vi "GetCtrlRef (String).vi"(8 "error in (no error)":errorcluster, 10 "FP Control":string, 11 "FP Controls in":refnum<class "FP Controls.lvclass">) -> (0 "error out":errorcluster, 2 "Ctrl Ref":refnum<vi>, 3 "FP Controls out":refnum<class "FP Controls.lvclass">)   [LabVIEW 2012, in "Configuration Grandmaster.lvlib" / "FP Controls.lvclass"]
uses:
  FP Controls.lvclass
  FP Controls.lvclass/FP Controls.ctl
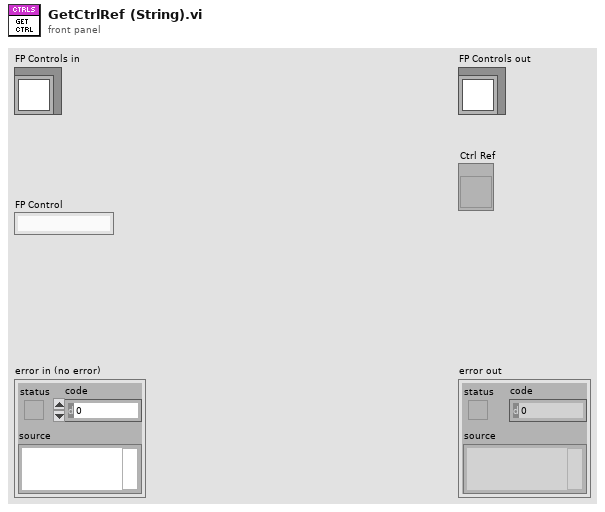
[diagram p1: front panel]
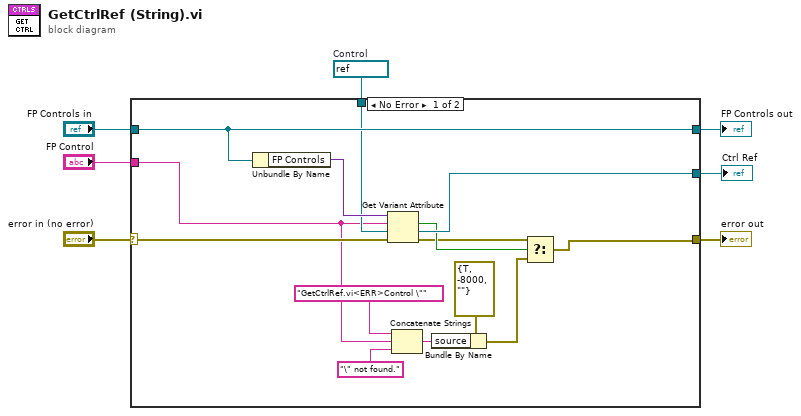
[diagram p0: block diagram]
diagram:
  w3 = refnum<vi> refnum  # Control
  n1 = case shown="No Error" "error in (no error)" {
    selector: "error in (no error)" -> [w9 w24]
    tunnel: [w15 w24] -> w6
    tunnel: [w21 w23] -> w4
    tunnel: "FP Controls in" -> [w21 w23]
    tunnel: w3 -> [w19 w22]
    tunnel: [w18 w22] -> w2
    tunnel: "FP Control" -> [w8 _]
    frame No Error {
      n2 = Unbundle By Name(w21) -> ("FP Controls"=w20:variant)
      n3 = Get Variant Attribute(Variant=w20, name=w8, default value (empty Variant)=w19, error in=w9) -> (found=w17:bool, value=w18:refnum<vi>, error out=w16:errorcluster)  [unwired: 1 out]
      n4 = Concatenate Strings("GetCtrlRef.vi<ERR>Control \"" ("source"), w8, "\" not found." ("source")) -> (w13:string)
      n5 = Bundle By Name(cluster=errorcluster {"status"=TRUE, "code"=-8000, "source"=""} ("error out"), "source"=w13) -> (w10:errorcluster)
      n6 = Select(t=w16, s=w17, f=w10) -> (s? t:f=w15:errorcluster)
    }
    frame Error {
    }
  }
  "error out" <- w6
  "FP Controls out" <- w4
  "Ctrl Ref" <- w2
